vi "Dialog.vi"(8 "error in (no error)":errorcluster, 11 "String":string) -> ()   [LabVIEW 2014]
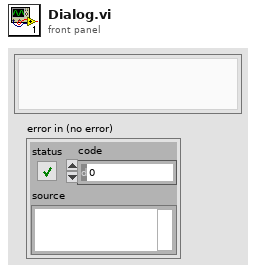
[diagram p1: front panel]
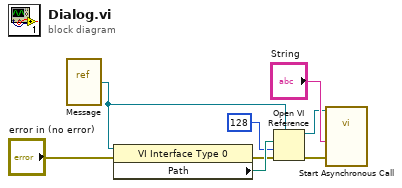
[diagram p0: block diagram]
diagram:
  n1 = vi-ref "Message.vi"() -> (w1:refnum<vi>)
  n2 = property class="VI Interface Type 0"(reference=w1, error in="error in (no error)") -> (error out=w5:errorcluster, "Path"=w7:path)  [unwired: 1 out]
  n3 = Open VI Reference(type specifier VI Refnum (for type only)=w1, vi path=w7, options=128, error in (no error)=w5) -> (vi reference=w3:refnum<vi>, error out=w2:errorcluster)  [unwired: 2 in]
  n4 = call-by-ref "Start Asynchronous Call"(reference=w3, "error in (no error)"=w2, "Message"="String") -> ()  [unwired: 9 in, 4 out]
